vi "Incorporate New Data.vi"(8 "error in (no error)":errorcluster, 10 "New Graph Data":waveform(dbl)[](array[waveform]), 11 "Data in":T1={"UI References"={"Exit Ref"=refnum, "Save Ref"=refnum, "Open Ref"=refnum, "Export Ref"=refnum, "Acquire Ref"=refnum, "Configure Ref"=refnum, "Graph Ref"=refnum, "Clear Ref"=refnum, "Analyze Ref"=refnum, "Status Ref"=refnum, "Snapshot Ref"=refnum}, "Graph Data"={"Data"=[], "Annotation List"=[], "Cursor List"=[], "Analysis Data"=[]}, "User Specified"={"Hardware Configuration"={"HW Refnum <Replace Me>"="", "Signal Type <Replace Me>"=enum."Sine Wave"}, "Analysis Configuration"={"Statistics"=TRUE}, "New Data Behavior"=enum."Replace"}}) -> (0 "error out":errorcluster, 3 "Data out":T1={"UI References"={"Exit Ref"=refnum, "Save Ref"=refnum, "Open Ref"=refnum, "Export Ref"=refnum, "Acquire Ref"=refnum, "Configure Ref"=refnum, "Graph Ref"=refnum, "Clear Ref"=refnum, "Analyze Ref"=refnum, "Status Ref"=refnum, "Snapshot Ref"=refnum}, "Graph Data"={"Data"=[], "Annotation List"=[], "Cursor List"=[], "Analysis Data"=[]}, "User Specified"={"Hardware Configuration"={"HW Refnum <Replace Me>"="", "Signal Type <Replace Me>"=enum."Sine Wave"}, "Analysis Configuration"={"Statistics"=TRUE}, "New Data Behavior"=enum."Replace"}})   [LabVIEW 2014]
doc: "Incorporates newly acquired or loaded data into the main state data. New data can replace, be appended to, or overlayed over (as an additional channel) existing data. If the user does not have a preference saved a dialog will be presented asking which method to use."
uses:
  controls/Data.ctl
  controls/UI References.ctl
  controls/Graph Data.ctl
  <vilib>/Utility/miscctls.llb/LVAnnotationListTypeDef.ctl
  <vilib>/Utility/miscctls.llb/LVCursorListTypeDef.ctl
  controls/User Specified Data.ctl
  controls/HW Configuration.ctl
  controls/Simulated Signal Type.ctl
  controls/Analysis Configuration.ctl
  controls/New Data Behavior.ctl
panel:
  # "(Scroll up to see large state data in/out clusters)"
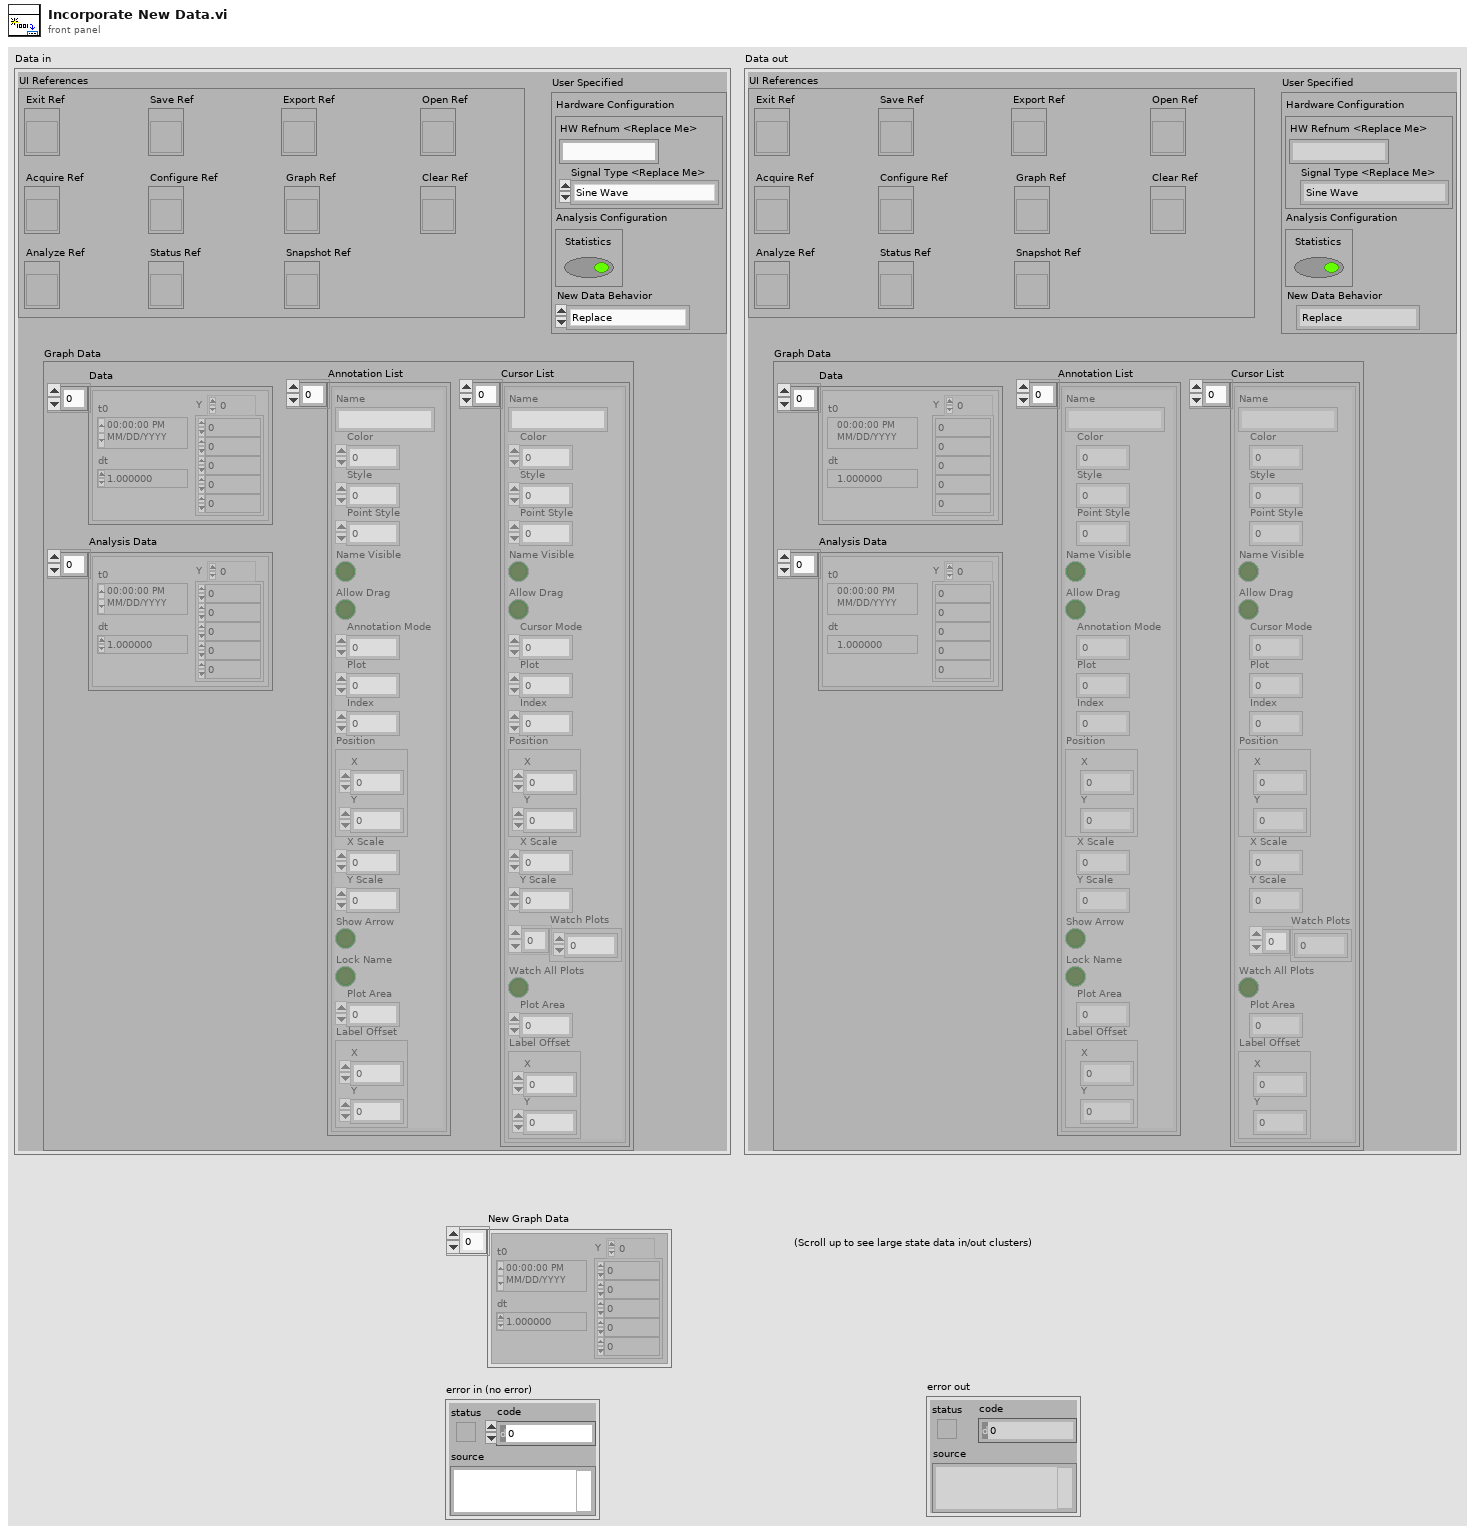
[diagram p1: front panel]
types:
  T1 = typedef "Data.ctl" = cluster{"UI References":T2, "Graph Data":T3, "User Specified":T6}
  T2 = typedef "UI References.ctl" = cluster{"Exit Ref":refnum<vi>, "Save Ref":refnum<vi>, "Open Ref":refnum<vi>, "Export Ref":refnum<vi>, "Acquire Ref":refnum<vi>, "Configure Ref":refnum<vi>, "Graph Ref":refnum<vi>, "Clear Ref":refnum<vi>, "Analyze Ref":refnum<vi>, "Status Ref":refnum<vi>, "Snapshot Ref":refnum<vi>}
  T3 = typedef "Graph Data.ctl" = cluster{"Data":waveform(dbl)[], "Annotation List":T4, "Cursor List":T5, "Analysis Data":waveform(dbl)[]}
  T4 = typedef "LVAnnotationListTypeDef.ctl" = cluster{"Name":string, "Color":u32, "Style":u8, "Point Style":u8, "Name Visible":bool, "Allow Drag":bool, "Annotation Mode":u32, "Plot":i32, "Index":i32, "Position":cluster{"X":dbl, "Y":dbl}, "X Scale":u32, "Y Scale":u32, "Show Arrow":bool, "Lock Name":bool, "Plot Area":i32, "Label Offset":cluster{"X":dbl, "Y":dbl}}[]
  T5 = typedef "LVCursorListTypeDef.ctl" = cluster{"Name":string, "Color":u32, "Style":u8, "Point Style":u8, "Name Visible":bool, "Allow Drag":bool, "Cursor Mode":u32, "Plot":i32, "Index":i32, "Position":cluster{"X":dbl, "Y":dbl}, "X Scale":u32, "Y Scale":u32, "Watch Plots":i32[], "Watch All Plots":bool, "Plot Area":i32, "Label Offset":cluster{"X":dbl, "Y":dbl}}[]
  T6 = typedef "User Specified Data.ctl" = cluster{"Hardware Configuration":T7, "Analysis Configuration":T9, "New Data Behavior":T10}
  T7 = typedef "HW Configuration.ctl" = cluster{"HW Refnum <Replace Me>":string, "Signal Type <Replace Me>":T8}
  T8 = typedef "Simulated Signal Type.ctl" = enum16{"Sine Wave", "Square Wave"}
  T9 = typedef "Analysis Configuration.ctl" = cluster{"Statistics":bool}
  T10 = typedef "New Data Behavior.ctl" = enum16{"Replace", "Overlay", "Append"}
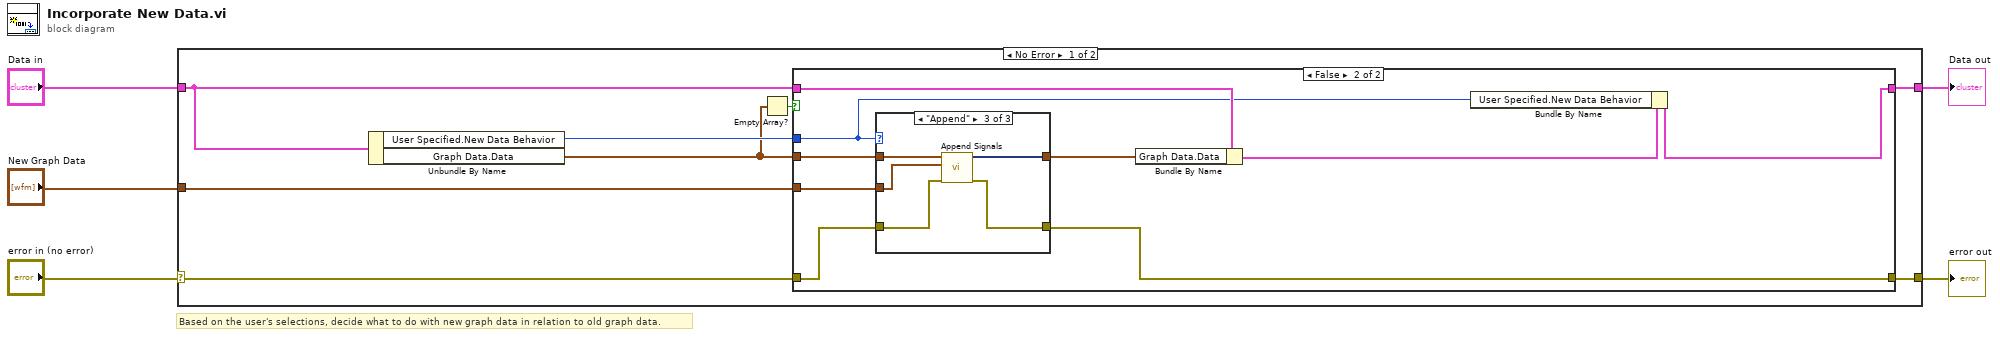
[diagram p0: block diagram]
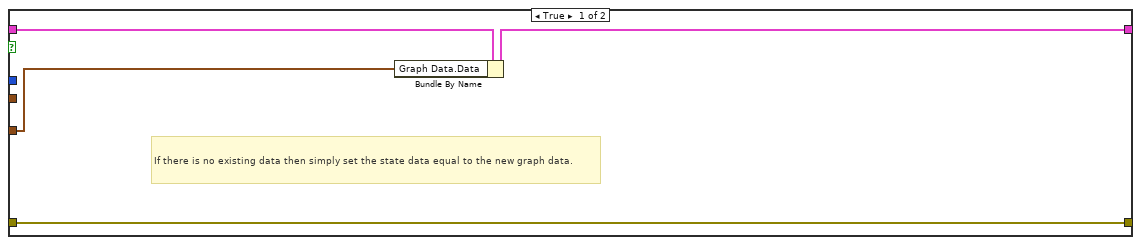
[diagram p2: hidden frame]
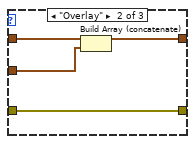
[diagram p4: hidden frame]
diagram:
  # "Based on the user's selections, decide what to do with new graph data in relation to old graph data."
  n1 = case shown="No Error" "error in (no error)" {
    selector: "error in (no error)" -> [w9 w39]
    tunnel: "Data in" -> [w13 w38]
    tunnel: "New Graph Data" -> [w11 _]
    tunnel: [w10 w38] -> w3
    tunnel: [w8 w39] -> w1
    frame No Error {
      n2 = Unbundle By Name(w13) -> ("User Specified.New Data Behavior"=w12:T10, "Graph Data.Data"=w7:waveform(dbl)[])
      n3 = Empty Array?(array=w7) -> (empty?=w6:bool)
      n4 = case shown="False" w6 {
        tunnel: w13 -> [w17 w26]
        tunnel: w12 -> [_ w18]
        tunnel: w11 -> [w16 w25]
        tunnel: w7 -> [_ w23]
        tunnel: [w15 w21] -> w10
        tunnel: w9 -> [w14 w20]
        tunnel: [w14 w19] -> w8
        frame True {
          # "If there is no existing data then simply set the state data equal to the new graph data."
          n5 = Bundle By Name(cluster=w17, "Graph Data.Data"=w16) -> (w15:T1)
        }
        frame False {
          n6 = case shown="\"Append\"" w18 {
            tunnel: w25 -> [w28 w31 w36]
            tunnel: [w28 w30 w35] -> w24
            tunnel: w23 -> [_ w32 w37]
            tunnel: w20 -> [w27 w29 w34]
            tunnel: [w27 w29 w33] -> w19
            frame "Replace" {
            }
            frame "Overlay" {
              n7 = Build Array (concatenate)(w32, w31) -> (w30:waveform(dbl)[])
            }
            frame "Append" {
              n8 = call "Append Signals"("error in (no error)"=w34, "Input Signal B"=w36, "Input Signal A"=w37) -> ("error out"=w33:errorcluster, "Appended Signals"=w35:dynamicdata)  [unwired: 7 in]
            }
          }
          n9 = Bundle By Name(cluster=w26, "Graph Data.Data"=w24) -> (w22:T1)
          n10 = Bundle By Name(cluster=w22, "User Specified.New Data Behavior"=w18) -> (w21:T1)
        }
      }
    }
    frame Error {
    }
  }
  "Data out" <- w3
  "error out" <- w1
